vi "Get Buffer.vi"(8 "error in (no error)":errorcluster, 11 "Carya Config (Buffer) in":refnum<class "CConfig By Ref Buffer.lvclass">) -> (0 "error out":errorcluster, 1 "Copy data?":bool=TRUE, 2 "Config":refnum<class "Carya Config.lvclass">, 3 "Carya Config (Buffer) out":refnum<class "CConfig By Ref Buffer.lvclass">)   [LabVIEW 2013, in "CConfig By Ref Buffer.lvclass"]
doc: "Copyright 2018, Carya Automatisering, Wiebe Walstra."
uses:
  CConfig By Ref Buffer.lvclass
  Carya Config.lvclass
  Buffer Functions.ctl
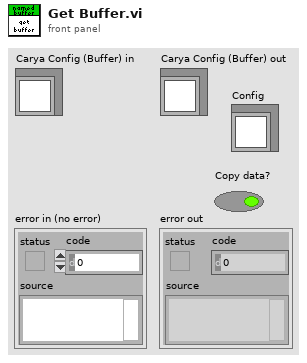
[diagram p1: front panel]
types:
  T1 = typedef "CConfig By Ref Buffer.lvclass/Buffer Functions.ctl" = enum16{"register", "get and lock", "set and unlock", "unlock", "unregister", "check"}
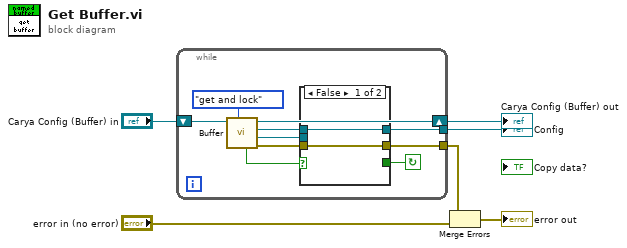
[diagram p0: block diagram]
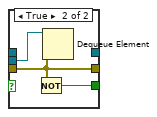
[diagram p2: hidden frame]
diagram:
  n1 = while {
    tunnel: [w12] -> w4
    shift-right: [w15] -> w5
    shift-left: "Carya Config (Buffer) in" -> [w16]
    tunnel: [w7] -> w1
    stop <- w8 continue-if-true
    n2 = call "Buffer.vi"("Functions"=Buffer_Functions."get and lock", "Carya Config (Buffer) in"=w16) -> ("error out"=w9:errorcluster, "queue out"=w13:refnum<queue>, "Config out"=w10:refnum<class "Carya Config.lvclass">, "Carya Config (Buffer) out"=w15:refnum<class "CConfig By Ref Buffer.lvclass">, "Wait\\Check"=w11:bool)  [unwired: 5 in]
    n3 = case shown="False" w11 {
      tunnel: w9 -> [w17 w19]
      tunnel: w13 -> [_ w21]
      tunnel: [w18 _] -> w12
      tunnel: w10 -> [w18 _]
      tunnel: [_ w20] -> w8
      tunnel: [w17 w19] -> w7
      frame False {
      }
      frame True {
        n4 = Not(x=w19) -> (.not. x?=w20:bool)
        n5 = Dequeue Element(queue=w21, error in (no error)=w19) -> ()  [unwired: 1 in, 4 out]
      }
    }
  }
  "Carya Config (Buffer) out" <- w5
  "Config" <- w4
  n6 = Merge Errors(w1, "error in (no error)") -> (→"error out":errorcluster)
